vi "topo_star.vi"(4 "deltat (TT-UT1)":dbl[unit], 5 "TimeStamp [UT1]":timestamp format="%<%H:%M:%S%6u\n%Y/%m/%d>T", 6 "error in (no error)":errorcluster, 7 "on_surface":T2 {"longitude" format="%_10g"; "latitude" format="%_10g"}, 8 "cat_entry":T1 {"dec" format="%.6g"; "ra" format="%.6g"}) -> (0 "error out":errorcluster, 3 "ra/dec":cluster{"ra":dbl[unit], "dec":dbl[unit]} {"dec" format="%_10g"; "ra" format="%_10g"})   [LabVIEW 2009]
uses:
  SiteInformation.ctl
  StarAstrometricEntry.ctl
  lib/novas-dll.dll
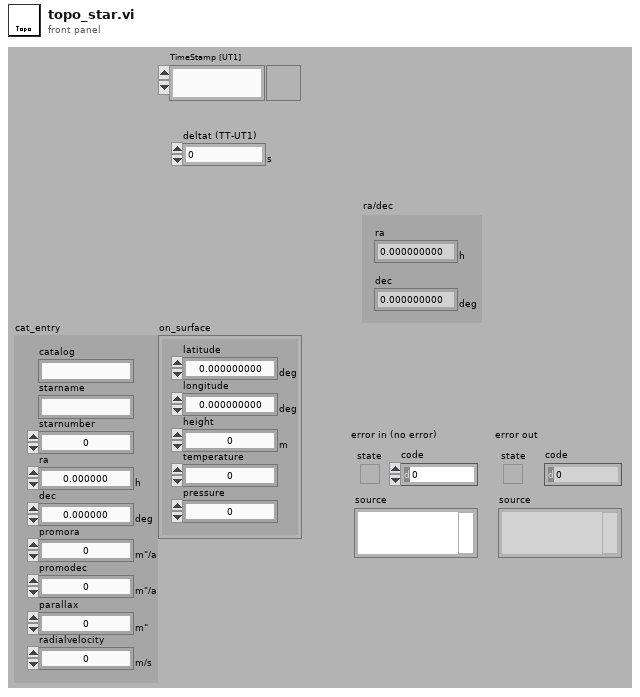
[diagram p1: front panel]
types:
  T1 = typedef "StarAstrometricEntry.ctl" = cluster{"catalog":string, "starname":string, "starnumber":i32, "ra":dbl[unit], "dec":dbl[unit], "promora":dbl[unit], "promodec":dbl[unit], "parallax":dbl[unit], "radialvelocity":dbl[unit]}
  T2 = typedef "SiteInformation.ctl" = cluster{"latitude":dbl[unit], "longitude":dbl[unit], "height":dbl[unit], "temperature":dbl, "pressure":dbl}
  T3 = cluster{"catalog":string, "starname":string, "starnumber":i32, "ra":dbl, "dec":dbl, "promora":dbl, "promodec":dbl, "parallax":dbl, "radialvelocity":dbl}
  T4 = cluster{"latitude":dbl, "longitude":dbl, "height":dbl, "temperature":dbl, "pressure":dbl}
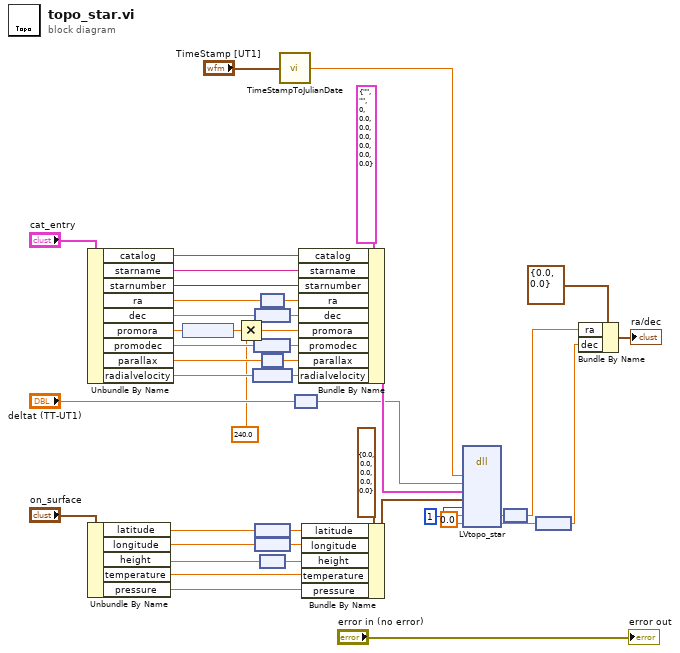
[diagram p0: block diagram]
diagram:
  w42 = 0.0 ("dec")
  n1 = Unbundle By Name("cat_entry") -> ("catalog"=w23:string, "starname"=w22:string, "starnumber"=w21:i32, "ra"=w20:dbl[unit], "dec"=w19:dbl[unit], "promora"=w7:dbl[unit], "promodec"=w18:dbl[unit], "parallax"=w17:dbl[unit], "radialvelocity"=w16:dbl[unit])
  n2 = Unbundle By Name("on_surface") -> ("latitude"=w38:dbl[unit], "longitude"=w37:dbl[unit], "height"=w36:dbl[unit], "temperature"=w35:dbl, "pressure"=w34:dbl)
  n3 = node(w7) -> (w6:dbl)
  n4 = Multiply(x=w6, y=240.0) -> (x*y=w4:dbl)
  n5 = node(w16) -> (w11:dbl)
  n6 = node(w18) -> (w13:dbl)
  n7 = node(w19) -> (w14:dbl)
  n8 = node(w38) -> (w31:dbl)
  n9 = node(w37) -> (w32:dbl)
  n10 = node(w36) -> (w33:dbl)
  n11 = node(w20) -> (w15:dbl)
  n12 = node(w17) -> (w12:dbl)
  n13 = call "TimeStampToJulianDate.vi"("TimeStamp [UT]"="TimeStamp [UT1]") -> ("JulianDay"=w3:ext)
  n14 = node("deltat (TT-UT1)") -> (w8:dbl)
  n15 = Bundle By Name(cluster=T3 {"catalog"="", "starname"="", "starnumber"=0, "ra"=0.0, "dec"=0.0, "promora"=0.0, "promodec"=0.0, "parallax"=0.0, "radialvelocity"=0.0} ("cat_entry"), "catalog"=w23, "starname"=w22, "starnumber"=w21, "ra"=w15, "dec"=w14, "promora"=w4, "promodec"=w13, "parallax"=w12, "radialvelocity"=w11) -> (w26:T3)
  n16 = Bundle By Name(cluster=T4 {"latitude"=0.0, "longitude"=0.0, "height"=0.0, "temperature"=0.0, "pressure"=0.0} ("site_info"), "latitude"=w31, "longitude"=w32, "height"=w33, "temperature"=w35, "pressure"=w34) -> (w39:T4)
  n17 = dll-call lib="C:/OhanaOS/Instruments/Novas/lib/novas-dll.dll" fn="LVtopo_star"("jd_tt"=w3, "delta_t"=w8, "star"=w26, "location"=w39, "accuracy"=i8 1, "ra"=w42, "dec"=w42) -> ("ra"=w43:dbl, "dec"=w44:dbl)  [unwired: 5 in, 6 out]
  n18 = node(w43) -> (w28:dbl[unit])
  n19 = node(w44) -> (w27:dbl[unit])
  n20 = Bundle By Name(cluster=cluster{"ra":dbl[unit], "dec":dbl[unit]} {"ra"=0.0, "dec"=0.0} ("ra/dec"), "ra"=w28, "dec"=w27) -> (→"ra/dec":cluster{"ra":dbl[unit], "dec":dbl[unit]})
  "error out" <- "error in (no error)"
